vi "DSPS_E36000.Get Current.vi"(8 "error in":errorcluster, 11 "VISA Alias":refnum<visa-resource-name>) -> (0 "error out":errorcluster, 1 "OC Trip":bool, 2 "Current":dbl, 3 "VISA Alias Dup":refnum<visa-resource-name>)   [LabVIEW 2018]
uses:
  <vilib>/KATE/Time/Time Utils.lvlib
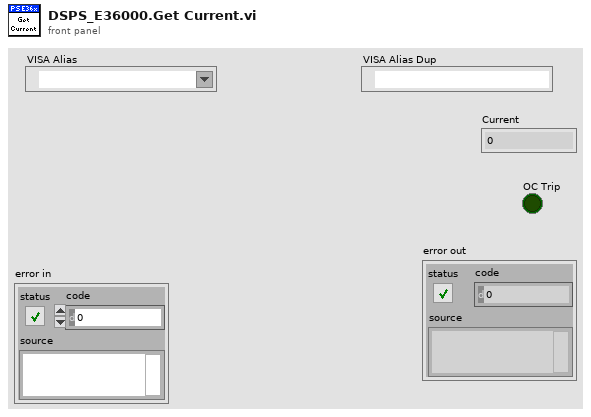
[diagram p1: front panel]
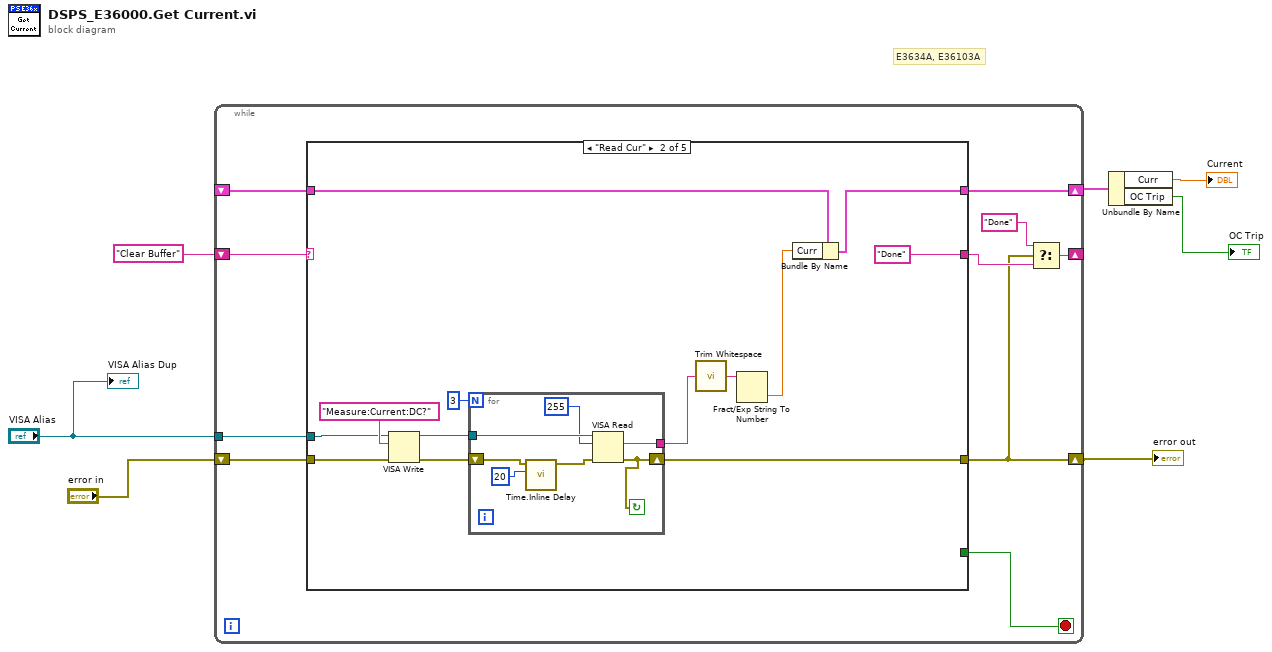
[diagram p0: block diagram]
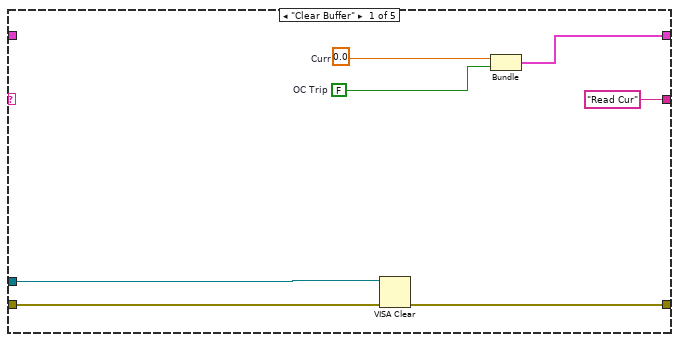
[diagram p2: hidden frame]
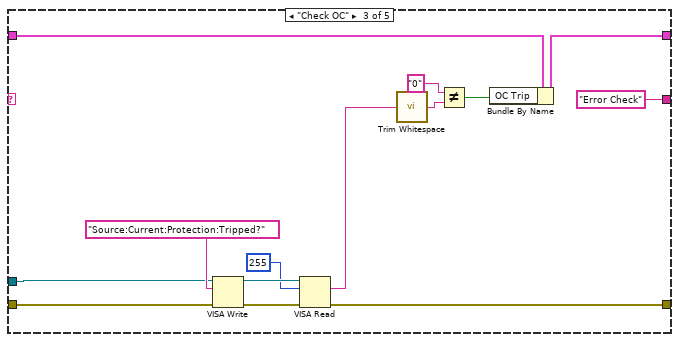
[diagram p3: hidden frame]
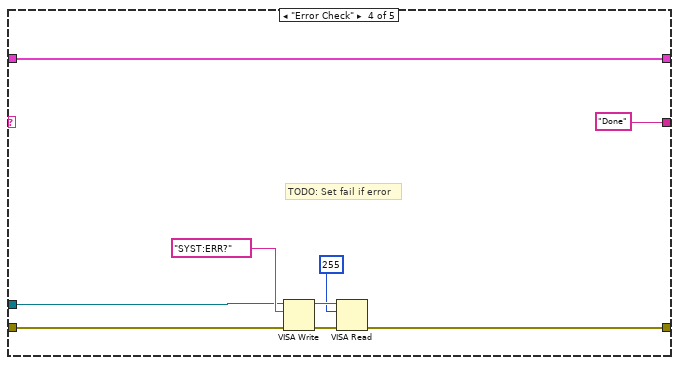
[diagram p4: hidden frame]
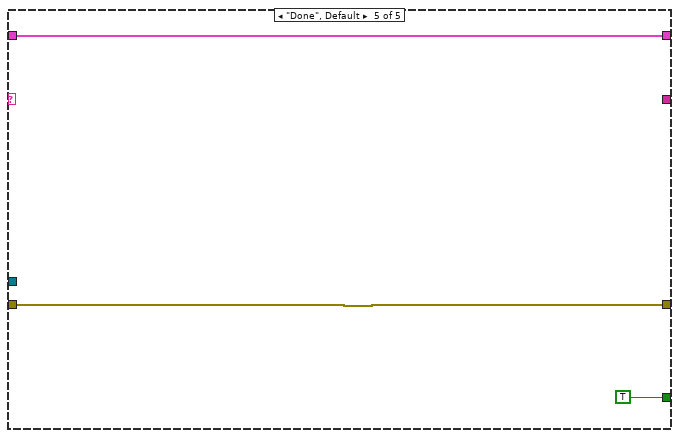
[diagram p5: hidden frame]
diagram:
  # "E3634A, E36103A"
  n1 = while {
    shift-right: [w13] -> w3
    shift-left: _ -> [w16]
    shift-right: [w10] -> _
    shift-left: "Clear Buffer" -> [w17]
    tunnel: "VISA Alias" -> [w15]
    shift-right: [w9] -> w4
    shift-left: "error in" -> [w14]
    stop <- w8 stop-if-true
    n2 = case shown="\"Read Cur\"" w17 {
      tunnel: w16 -> [_ w33 w54 w60 w69]
      tunnel: w15 -> [w20 w36 w57 w63 _]
      tunnel: w14 -> [w19 w35 w56 w61 w68]
      tunnel: [w18 w30 w50 w62 w68] -> w9
      tunnel: [w24 w32 w53 w60 w69] -> w13
      tunnel: ["Read Cur" "Done" "Error Check" "Done" _] -> w11
      tunnel: [_ _ _ _ TRUE] -> w8
      frame "Clear Buffer" {
        w21 = FALSE  # OC Trip
        w22 = 0.0  # Curr
        n3 = VISA Clear(VISA resource name=w20, error in (no error)=w19) -> (error out=w18:errorcluster)  [unwired: 1 out]
        n4 = Bundle("Curr"=w22, "OC Trip"=w21) -> (w24:cluster{"Curr":dbl, "OC Trip":bool})  [unwired: 1 in]
      }
      frame "Read Cur" {
        n5 = VISA Write(VISA resource name=w36, write buffer="Measure:Current:DC?", error in (no error)=w35) -> (VISA resource name out=w31:refnum<visa-resource-name>, error out=w26:errorcluster)  [unwired: 1 out]
        n6 = for {
          N: 3 -> [_]
          tunnel: w31 -> [w44]
          tunnel: [w42] -> w29
          shift-right: [w38] -> w30
          shift-left: w26 -> [w41]
          stop <- w38 continue-if-true
          n7 = call <vilib>:"Time.Inline Delay.vi"("Wait(ms)"=u32 20, "error in top"=w41) -> ("error out top"=w40:errorcluster)  [unwired: 8 in, 1 out]
          n8 = VISA Read(VISA resource name=w44, byte count=u32 255, error in (no error)=w40) -> (read buffer=w42:string, error out=w38:errorcluster)  [unwired: 2 out]
        }
        n9 = call <vilib>:"Trim Whitespace.vi"("string"=w29) -> ("trimmed string"=w28:string)  [unwired: 1 in]
        n10 = Fract/Exp String To Number(string=w28) -> (number=w27:dbl)  [unwired: 3 in, 1 out]
        n11 = Bundle By Name(cluster=w33, "Curr"=w27) -> (w32:cluster{"Curr":dbl, "OC Trip":bool})
      }
      frame "Check OC" {
        n12 = VISA Write(VISA resource name=w57, write buffer="Source:Current:Protection:Tripped?", error in (no error)=w56) -> (VISA resource name out=w52:refnum<visa-resource-name>, error out=w51:errorcluster)  [unwired: 1 out]
        n13 = VISA Read(VISA resource name=w52, byte count=u32 255, error in (no error)=w51) -> (read buffer=w46:string, error out=w50:errorcluster)  [unwired: 2 out]
        n14 = call <vilib>:"Trim Whitespace.vi"("string"=w46) -> ("trimmed string"=w48:string)  [unwired: 1 in]
        n15 = Not Equal?(x="0", y=w48) -> (x != y?=w49:bool)
        n16 = Bundle By Name(cluster=w54, "OC Trip"=w49) -> (w53:cluster{"Curr":dbl, "OC Trip":bool})
      }
      frame "Error Check" {
        # "TODO: Set fail if error"
        n17 = VISA Write(VISA resource name=w63, write buffer="SYST:ERR?", error in (no error)=w61) -> (VISA resource name out=w67:refnum<visa-resource-name>, error out=w65:errorcluster)  [unwired: 1 out]
        n18 = VISA Read(VISA resource name=w67, byte count=u32 255 ("byte count (0)"), error in (no error)=w65) -> (error out=w62:errorcluster)  [unwired: 3 out]
      }
      frame "Done", Default {
      }
    }
    n19 = Select(t="Done", s=w9, f=w11) -> (s? t:f=w10:string)
  }
  "error out" <- w4
  n20 = Unbundle By Name(w3) -> ("Curr"=→"Current":dbl, "OC Trip"=→"OC Trip":bool)
  "VISA Alias Dup" <- "VISA Alias"
